vi "002_1337Tubes.vi"() -> ()   [LabVIEW 2010]
panel:
  out "Numeric":dbl
  out "String":string
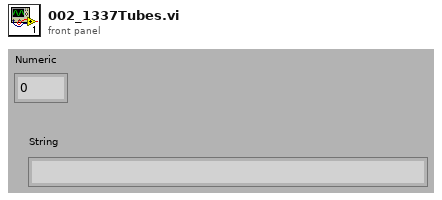
[diagram p1: front panel]
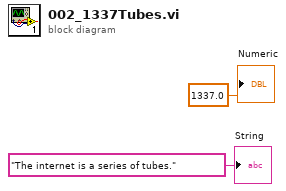
[diagram p0: block diagram]
diagram:
  "String" <- "The internet is a series of tubes." ("String")
  "Numeric" <- 1337.0 ("Numeric")
